vi "Update_Result_Table.vi"(7 "MCListbox Refnum":refnum<vi>, 9 "TempAnalysisResult":variant, 10 "ProjectName":string, 11 "Analysis Result":refnum<vi>) -> ()   [LabVIEW 2019]
uses:
  ROI/Controls/ROI_List_Action.ctl
  Analysis/Controls/Parttern Match/Analysis_PatternMatch_Parameter.ctl
  Analysis/Controls/Barcode 1D/Analysis_Barcode 1D_Parameter.ctl
  <vilib>/vision/Instrument.llb/Demodulation Mode.ctl
  <vilib>/vision/Instrument.llb/Cell Sample Size.ctl
  <vilib>/vision/Instrument.llb/Cell Filter Mode.ctl
  <vilib>/vision/Instrument.llb/QR Code Search Options.ctl
  <vilib>/vision/Instrument.llb/Data Matrix Polarity.ctl
  <vilib>/vision/Instrument.llb/QR Code Model Type.ctl
  <vilib>/vision/Instrument.llb/QR Code Description Options.ctl
  Analysis/Controls/Barcode 2D/Analysis_Barcode 2D_Parameter.ctl
  Analysis/Controls/Clamp MAX/Analysis_Clamp MAX_Parameter.ctl
  Analysis/Controls/Clamp/Analysis_Clamp_Parameter.ctl
  Analysis/Controls/Edge Detection/Analysis_Edge Detection_Parameter.ctl
  Analysis/Controls/Find Straight Edge/Analysis_Find Straight Edge_Parameter.ctl
  <vilib>/vision/Measure.llb/Straight Edge Process.ctl
  <vilib>/vision/Measure.llb/Straight Edge Options.ctl
  <vilib>/vision/Measure.llb/Edge Polarity.ctl
  <vilib>/vision/Measure.llb/Edge Options.ctl
  <vilib>/vision/Instrument.llb/Data Matrix Search Options.ctl
  <vilib>/vision/Instrument.llb/Data Matrix Mirror.ctl
  <vilib>/vision/Instrument.llb/Cell Fill Percentage.ctl
  <vilib>/vision/Instrument.llb/ECC Type.ctl
  <vilib>/vision/Instrument.llb/Data Matrix Description Options.ctl
  Analysis/Controls/Particle/Analysis_Particle_Parameter.ctl
  Analysis/Controls/Histogram/Analysis_Histogram_Parameter.ctl
  Analysis/Controls/Circle/Analysis_Circle_Parameter.ctl
  Analysis/Controls/ShapeDectect/Analysis_ShapeDectect_Parameter.ctl
  Analysis/Controls/OCR/Analysis_OCR_Setting Parameter.ctl
  Analysis/Controls/ColorMatch/Analysis_ColorMatch_Parameter.ctl
  <vilib>/vision/Instrument.llb/Data Matrix Advanced Options.ctl
  <vilib>/vision/Instrument.llb/Data Matrix Size Options.ctl
panel:
  in  "Selected Particle Report":T1(array[cluster])=[{"Area"=25.0, "Number of Holes"=0.0, "Bounding Rect"={"Left"=86.0, "Top"=0.0, "Right"=95.0, "Bottom"=7.0}, "Center of Mass"={"X"=89.88, "Y"=2.56}, "Orientation"=35.64802944169076, "Dimensions"={"Width"=9.0, "Height"=7.0}}, {"Area"=86262.0, "Number of Holes"=23.0, "Bounding Rect"={"Left"=0.0, "Top"=0.0, "Right"=463.0, "Bottom"=400.0}, "Center of Mass"={"X"=231.6348565996615, "Y"=215.4975423709165}, "Orientation"=163.33264135410136, "Dimensions"={"Width"=463.0, "Height"=400.0}}, {"Area"=1.0, "Number of Holes"=0.0, "Bounding Rect"={"Left"=412.0, "Top"=1.0, "Right"=413.0, "Bottom"=2.0}, "Center of Mass"={"X"=412.0, "Y"=1.0}, "Orientation"=-0.0, "Dimensions"={"Width"=1.0, "Height"=1.0}}, {"Area"=764.0, "Number of Holes"=1.0, "Bounding Rect"={"Left"=400.0, "Top"=1.0, "Right"=429.0, "Bottom"=38.0}, "Center of Mass"={"X"=414.1609947643979, "Y"=19.994764397905758}, "Orientation"=91.15464026101695, "Dimensions"={"Width"=29.0, "Height"=37.0}}, {"Area"=59.0, "Number of Holes"=0.0, "Bounding Rect"={"Left"=310.0, "Top"=6.0, "Right"=340.0, "Bottom"=29.0}, "Center of Mass"={"X"=326.50847457627117, "Y"=15.610169491525424}, "Orientation"=141.9692279302436, "Dimensions"={"Width"=30.0, "Height"=23.0}}, {"Area"=11.0, "Number of Holes"=0.0, "Bounding Rect"={"Left"=0.0, "Top"=7.0, "Right"=8.0, "Bottom"=12.0}, "Center of Mass"={"X"=3.090909090909091, "Y"=9.0}, "Orientation"=154.0962999034186, "Dimensions"={"Width"=8.0, "Height"=5.0}}, {"Area"=8.0, "Number of Holes"=0.0, "Bounding Rect"={"Left"=10.0, "Top"=12.0, "Right"=18.0, "Bottom"=15.0}, "Center of Mass"={"X"=13.5, "Y"=13.125}, "Orientation"=161.9863133074482, "Dimensions"={"Width"=8.0, "Height"=3.0}}, {"Area"=2191.0, "Number of Holes"=0.0, "Bounding Rect"={"Left"=108.0, "Top"=12.0, "Right"=160.0, "Bottom"=73.0}, "Center of Mass"={"X"=132.4596074851666, "Y"=44.30716567777271}, "Orientation"=94.97370367521454, "Dimensions"={"Width"=52.0, "Height"=61.0}}, {"Area"=18.0, "Number of Holes"=0.0, "Bounding Rect"={"Left"=136.0, "Top"=12.0, "Right"=150.0, "Bottom"=18.0}, "Center of Mass"={"X"=142.94444444444446, "Y"=13.833333333333334}, "Orientation"=159.1562056734768, "Dimensions"={"Width"=14.0, "Height"=6.0}}, {"Area"=4659.0, "Number of Holes"=2.0, "Bounding Rect"={"Left"=266.0, "Top"=12.0, "Right"=345.0, "Bottom"=101.0}, "Center of Mass"={"X"=303.5157759175789, "Y"=58.89869070616012}, "Orientation"=93.68626534635163, "Dimensions"={"Width"=79.0, "Height"=89.0}}, {"Area"=12.0, "Number of Holes"=0.0, "Bounding Rect"={"Left"=19.0, "Top"=14.0, "Right"=29.0, "Bottom"=17.0}, "Center of Mass"={"X"=23.083333333333332, "Y"=15.416666666666666}, "Orientation"=169.41797481154816, "Dimensions"={"Width"=10.0, "Height"=3.0}}, {"Area"=6.0, "Number of Holes"=0.0, "Bounding Rect"={"Left"=32.0, "Top"=17.0, "Right"=38.0, "Bottom"=18.0}, "Center of Mass"={"X"=34.5, "Y"=17.0}, "Orientation"=-0.0, "Dimensions"={"Width"=6.0, "Height"=1.0}}, {"Area"=1.0, "Number of Holes"=0.0, "Bounding Rect"={"Left"=40.0, "Top"=17.0, "Right"=41.0, "Bottom"=18.0}, "Center of Mass"={"X"=40.0, "Y"=17.0}, "Orientation"=-0.0, "Dimensions"={"Width"=1.0, "Height"=1.0}}, {"Area"=1.0, "Number of Holes"=0.0, "Bounding Rect"={"Left"=326.0, "Top"=23.0, "Right"=327.0, "Bottom"=24.0}, "Center of Mass"={"X"=326.0, "Y"=23.0}, "Orientation"=-0.0, "Dimensions"={"Width"=1.0, "Height"=1.0}}, {"Area"=72.0, "Number of Holes"=2.0, "Bounding Rect"={"Left"=388.0, "Top"=35.0, "Right"=410.0, "Bottom"=55.0}, "Center of Mass"={"X"=397.8888888888889, "Y"=46.52777777777778}, "Orientation"=136.8853757704328, "Dimensions"={"Width"=22.0, "Height"=20.0}}, {"Area"=2.0, "Number of Holes"=0.0, "Bounding Rect"={"Left"=342.0, "Top"=36.0, "Right"=343.0, "Bottom"=38.0}, "Center of Mass"={"X"=342.0, "Y"=36.5}, "Orientation"=90.0, "Dimensions"={"Width"=1.0, "Height"=2.0}}, {"Area"=1.0, "Number of Holes"=0.0, "Bounding Rect"={"Left"=396.0, "Top"=49.0, "Right"=397.0, "Bottom"=50.0}, "Center of Mass"={"X"=396.0, "Y"=49.0}, "Orientation"=-0.0, "Dimensions"={"Width"=1.0, "Height"=1.0}}, {"Area"=2.0, "Number of Holes"=0.0, "Bounding Rect"={"Left"=411.0, "Top"=54.0, "Right"=413.0, "Bottom"=55.0}, "Center of Mass"={"X"=411.5, "Y"=54.0}, "Orientation"=-0.0, "Dimensions"={"Width"=2.0, "Height"=1.0}}, {"Area"=86.0, "Number of Holes"=0.0, "Bounding Rect"={"Left"=457.0, "Top"=74.0, "Right"=463.0, "Bottom"=96.0}, "Center of Mass"={"X"=460.2674418604651, "Y"=84.55813953488372}, "Orientation"=89.65892383367937, "Dimensions"={"Width"=6.0, "Height"=22.0}}, {"Area"=1300.0, "Number of Holes"=0.0, "Bounding Rect"={"Left"=30.0, "Top"=82.0, "Right"=67.0, "Bottom"=127.0}, "Center of Mass"={"X"=48.050769230769234, "Y"=104.12153846153846}, "Orientation"=84.17144755534598, "Dimensions"={"Width"=37.0, "Height"=45.0}}, {"Area"=1.0, "Number of Holes"=0.0, "Bounding Rect"={"Left"=450.0, "Top"=105.0, "Right"=451.0, "Bottom"=106.0}, "Center of Mass"={"X"=450.0, "Y"=105.0}, "Orientation"=-0.0, "Dimensions"={"Width"=1.0, "Height"=1.0}}, {"Area"=3.0, "Number of Holes"=0.0, "Bounding Rect"={"Left"=243.0, "Top"=124.0, "Right"=245.0, "Bottom"=126.0}, "Center of Mass"={"X"=243.66666666666666, "Y"=124.33333333333333}, "Orientation"=135.00000000000014, "Dimensions"={"Width"=2.0, "Height"=2.0}}, {"Area"=28.0, "Number of Holes"=0.0, "Bounding Rect"={"Left"=271.0, "Top"=127.0, "Right"=293.0, "Bottom"=136.0}, "Center of Mass"={"X"=281.39285714285717, "Y"=131.39285714285714}, "Orientation"=158.88118737593115, "Dimensions"={"Width"=22.0, "Height"=9.0}}, {"Area"=4.0, "Number of Holes"=0.0, "Bounding Rect"={"Left"=250.0, "Top"=128.0, "Right"=253.0, "Bottom"=130.0}, "Center of Mass"={"X"=251.0, "Y"=128.5}, "Orientation"=148.282525588539, "Dimensions"={"Width"=3.0, "Height"=2.0}}, {"Area"=4.0, "Number of Holes"=0.0, "Bounding Rect"={"Left"=255.0, "Top"=132.0, "Right"=258.0, "Bottom"=134.0}, "Center of Mass"={"X"=256.0, "Y"=132.5}, "Orientation"=148.282525588539, "Dimensions"={"Width"=3.0, "Height"=2.0}}, {"Area"=2.0, "Number of Holes"=0.0, "Bounding Rect"={"Left"=260.0, "Top"=136.0, "Right"=262.0, "Bottom"=138.0}, "Center of Mass"={"X"=260.5, "Y"=136.5}, "Orientation"=135.0, "Dimensions"={"Width"=2.0, "Height"=2.0}}, {"Area"=1.0, "Number of Holes"=0.0, "Bounding Rect"={"Left"=300.0, "Top"=136.0, "Right"=301.0, "Bottom"=137.0}, "Center of Mass"={"X"=300.0, "Y"=136.0}, "Orientation"=-0.0, "Dimensions"={"Width"=1.0, "Height"=1.0}}, {"Area"=6.0, "Number of Holes"=0.0, "Bounding Rect"={"Left"=263.0, "Top"=139.0, "Right"=269.0, "Bottom"=145.0}, "Center of Mass"={"X"=265.5, "Y"=141.5}, "Orientation"=135.0, "Dimensions"={"Width"=6.0, "Height"=6.0}}, {"Area"=4.0, "Number of Holes"=0.0, "Bounding Rect"={"Left"=296.0, "Top"=139.0, "Right"=299.0, "Bottom"=141.0}, "Center of Mass"={"X"=297.25, "Y"=139.25}, "Orientation"=161.56505117707798, "Dimensions"={"Width"=3.0, "Height"=2.0}}, {"Area"=1.0, "Number of Holes"=0.0, "Bounding Rect"={"Left"=269.0, "Top"=146.0, "Right"=270.0, "Bottom"=147.0}, "Center of Mass"={"X"=269.0, "Y"=146.0}, "Orientation"=-0.0, "Dimensions"={"Width"=1.0, "Height"=1.0}}, {"Area"=3.0, "Number of Holes"=0.0, "Bounding Rect"={"Left"=271.0, "Top"=148.0, "Right"=273.0, "Bottom"=151.0}, "Center of Mass"={"X"=271.3333333333333, "Y"=149.0}, "Orientation"=118.15496623701016, "Dimensions"={"Width"=2.0, "Height"=3.0}}, {"Area"=2795.0, "Number of Holes"=2.0, "Bounding Rect"={"Left"=375.0, "Top"=149.0, "Right"=427.0, "Bottom"=220.0}, "Center of Mass"={"X"=400.8608228980322, "Y"=184.37352415026834}, "Orientation"=84.46336335814708, "Dimensions"={"Width"=52.0, "Height"=71.0}}, {"Area"=6024.0, "Number of Holes"=9.0, "Bounding Rect"={"Left"=176.0, "Top"=152.0, "Right"=254.0, "Bottom"=252.0}, "Center of Mass"={"X"=211.63097609561754, "Y"=201.42861885790174}, "Orientation"=84.84991716022375, "Dimensions"={"Width"=78.0, "Height"=100.0}}, {"Area"=1.0, "Number of Holes"=0.0, "Bounding Rect"={"Left"=275.0, "Top"=154.0, "Right"=276.0, "Bottom"=155.0}, "Center of Mass"={"X"=275.0, "Y"=154.0}, "Orientation"=-0.0, "Dimensions"={"Width"=1.0, "Height"=1.0}}, {"Area"=2.0, "Number of Holes"=0.0, "Bounding Rect"={"Left"=462.0, "Top"=209.0, "Right"=463.0, "Bottom"=211.0}, "Center of Mass"={"X"=462.0, "Y"=209.5}, "Orientation"=90.0, "Dimensions"={"Width"=1.0, "Height"=2.0}}, {"Area"=1.0, "Number of Holes"=0.0, "Bounding Rect"={"Left"=460.0, "Top"=214.0, "Right"=461.0, "Bottom"=215.0}, "Center of Mass"={"X"=460.0, "Y"=214.0}, "Orientation"=-0.0, "Dimensions"={"Width"=1.0, "Height"=1.0}}, {"Area"=2.0, "Number of Holes"=0.0, "Bounding Rect"={"Left"=459.0, "Top"=216.0, "Right"=460.0, "Bottom"=218.0}, "Center of Mass"={"X"=459.0, "Y"=216.5}, "Orientation"=90.0, "Dimensions"={"Width"=1.0, "Height"=2.0}}, {"Area"=3.0, "Number of Holes"=0.0, "Bounding Rect"={"Left"=249.0, "Top"=220.0, "Right"=251.0, "Bottom"=223.0}, "Center of Mass"={"X"=249.66666666666666, "Y"=221.0}, "Orientation"=61.84503376298985, "Dimensions"={"Width"=2.0, "Height"=3.0}}, {"Area"=1243.0, "Number of Holes"=2.0, "Bounding Rect"={"Left"=26.0, "Top"=222.0, "Right"=62.0, "Bottom"=266.0}, "Center of Mass"={"X"=43.17940466613033, "Y"=243.51729686242962}, "Orientation"=85.94368880614128, "Dimensions"={"Width"=36.0, "Height"=44.0}}, {"Area"=3.0, "Number of Holes"=0.0, "Bounding Rect"={"Left"=248.0, "Top"=224.0, "Right"=250.0, "Bottom"=227.0}, "Center of Mass"={"X"=248.33333333333334, "Y"=225.0}, "Orientation"=61.84503376298985, "Dimensions"={"Width"=2.0, "Height"=3.0}}, {"Area"=1.0, "Number of Holes"=0.0, "Bounding Rect"={"Left"=62.0, "Top"=237.0, "Right"=63.0, "Bottom"=238.0}, "Center of Mass"={"X"=62.0, "Y"=237.0}, "Orientation"=-0.0, "Dimensions"={"Width"=1.0, "Height"=1.0}}, {"Area"=1.0, "Number of Holes"=0.0, "Bounding Rect"={"Left"=63.0, "Top"=241.0, "Right"=64.0, "Bottom"=242.0}, "Center of Mass"={"X"=63.0, "Y"=241.0}, "Orientation"=-0.0, "Dimensions"={"Width"=1.0, "Height"=1.0}}, {"Area"=25.0, "Number of Holes"=0.0, "Bounding Rect"={"Left"=60.0, "Top"=277.0, "Right"=78.0, "Bottom"=285.0}, "Center of Mass"={"X"=68.52, "Y"=279.96}, "Orientation"=21.66201240397291, "Dimensions"={"Width"=18.0, "Height"=8.0}}, {"Area"=2.0, "Number of Holes"=0.0, "Bounding Rect"={"Left"=57.0, "Top"=285.0, "Right"=59.0, "Bottom"=287.0}, "Center of Mass"={"X"=57.5, "Y"=285.5}, "Orientation"=45.0, "Dimensions"={"Width"=2.0, "Height"=2.0}}, {"Area"=1575.0, "Number of Holes"=0.0, "Bounding Rect"={"Left"=302.0, "Top"=285.0, "Right"=345.0, "Bottom"=337.0}, "Center of Mass"={"X"=321.4095238095238, "Y"=308.74603174603175}, "Orientation"=73.7943685874199, "Dimensions"={"Width"=43.0, "Height"=52.0}}, {"Area"=4853.0, "Number of Holes"=6.0, "Bounding Rect"={"Left"=54.0, "Top"=304.0, "Right"=130.0, "Bottom"=388.0}, "Center of Mass"={"X"=91.93962497424273, "Y"=344.35854110859265}, "Orientation"=86.14198788768665, "Dimensions"={"Width"=76.0, "Height"=84.0}}, {"Area"=28.0, "Number of Holes"=0.0, "Bounding Rect"={"Left"=323.0, "Top"=332.0, "Right"=338.0, "Bottom"=341.0}, "Center of Mass"={"X"=330.57142857142856, "Y"=336.64285714285717}, "Orientation"=29.47782205630064, "Dimensions"={"Width"=15.0, "Height"=9.0}}, {"Area"=3.0, "Number of Holes"=0.0, "Bounding Rect"={"Left"=312.0, "Top"=366.0, "Right"=315.0, "Bottom"=367.0}, "Center of Mass"={"X"=313.0, "Y"=366.0}, "Orientation"=-0.0, "Dimensions"={"Width"=3.0, "Height"=1.0}}, {"Area"=1.0, "Number of Holes"=0.0, "Bounding Rect"={"Left"=436.0, "Top"=396.0, "Right"=437.0, "Bottom"=397.0}, "Center of Mass"={"X"=436.0, "Y"=396.0}, "Orientation"=-0.0, "Dimensions"={"Width"=1.0, "Height"=1.0}}, {"Area"=1.0, "Number of Holes"=0.0, "Bounding Rect"={"Left"=434.0, "Top"=397.0, "Right"=435.0, "Bottom"=398.0}, "Center of Mass"={"X"=434.0, "Y"=397.0}, "Orientation"=-0.0, "Dimensions"={"Width"=1.0, "Height"=1.0}}, {"Area"=36.0, "Number of Holes"=0.0, "Bounding Rect"={"Left"=318.0, "Top"=398.0, "Right"=340.0, "Bottom"=400.0}, "Center of Mass"={"X"=328.5, "Y"=398.6111111111111}, "Orientation"=-0.0, "Dimensions"={"Width"=22.0, "Height"=2.0}}, {"Area"=8.0, "Number of Holes"=0.0, "Bounding Rect"={"Left"=427.0, "Top"=398.0, "Right"=433.0, "Bottom"=400.0}, "Center of Mass"={"X"=429.75, "Y"=398.625}, "Orientation"=11.525650458236512, "Dimensions"={"Width"=6.0, "Height"=2.0}}]
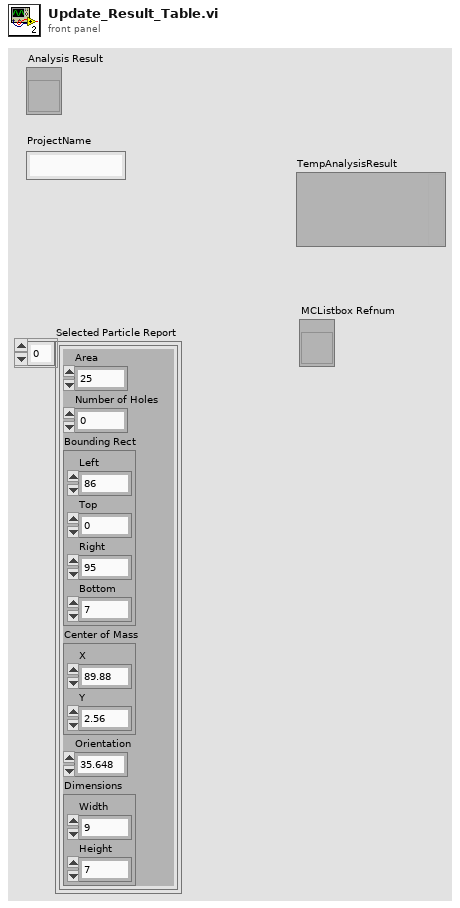
[diagram p1: front panel]
types:
  T1 = cluster{"Area":dbl, "Number of Holes":dbl, "Bounding Rect":cluster{"Left":dbl, "Top":dbl, "Right":dbl, "Bottom":dbl}, "Center of Mass":cluster{"X":dbl, "Y":dbl}, "Orientation":dbl, "Dimensions":cluster{"Width":dbl, "Height":dbl}}[]
  T2 = typedef "ROI_List_Action.ctl" = enum16{"Init", "Add ROI", "Delete ROI", "Get All ROI", "Get Specific ROI", "Set Analysis Setting", "Set Process Setting", "Replace All Entries", "ROIEntryBackup", "ROIEntryBackupClear", "ROIEntryReturn"}
  T3 = typedef "Vision_DataEntry.ctl" = cluster{"vROIName":string, "vROIContour":cluster{"Contour Type":u32, "ROI Type":u32, "Points":i32[]}, "ProcessSetting":T4[], "Analysis_Setting":T6}
  T4 = typedef "Process_Setting.ctl" = cluster{"Enum_PreProcess":T5, "Parameter":string}
  T5 = typedef "VisionProcessName.ctl" = enum16{"*CamParameter*", "CamAttributes", "*Preprocess*", "CG_Brightness", "C_Plane Extraction", "C_Threshold", "G_Lookup Table", "G_Threshold"}
  T6 = typedef "Analysis_Setting.ctl" = cluster{"PreProcess":T7, "Parameter":string}
  T7 = typedef "V_Analysis_Type.ctl" = enum16{"None", "C_Color Pattern Matching", "G_PatternMatching", "G_ShapeDectect", "G_GeometricMatch", "B_Area Check"}
  T8 = typedef "ROI Descriptor" = cluster{"Global Rectangle":i32[], "Contours":cluster{"ID":enum32{"External", "Internal"}, "Type":u32, "Coordinates":i32[]}[]}
  T9 = cluster{"Algorithm":i32, "Match Parameters":cluster{"Number of Matches Requested":i32, "Minimum Match Score":sgl, "Angle Ranges":cluster{"Start Angle":sgl, "End Angle":sgl}[]}, "ROI Descriptor":T8, "Advanced Options":cluster{"Item":u16, "Value":dbl}[], "Template path":string}
  T10 = typedef "Analysis_Circle_Parameter.ctl" = cluster{"ROI Descriptor":cluster{"Global Rectangle":i32[], "Contours":cluster{"Contour Type":u32, "ROI Type":u32, "Points":i32[]}[]}, "Options":cluster{"Search  Direction":u32, "Edge Options":T11, "Show Search Area":bool, "Show Search Lines":bool, "Show Edges Found":bool, "Show Result":bool, "Search Area Color":u32, "Search Lines Color":u32, "Edge Locations Color":u32, "Result Color":u32, "Overlay Group Name":string}, "Circle Fit Options":cluster{"Process":enum16{"Get First Edge", "Get First + Last Edge", "Get All Edges", "Get Best Edge"}, "Step Size":dbl, "Max Pixel Radius":i32}}
  T11 = typedef "Edge Options.ctl" = cluster{"Edge Polarity":T12, "Kernel Size":u32, "Width":u32, "Minimum Edge Strength":sgl, "Interpolation Type":enum32{"Zero Order", "Bilinear", "Quadratic", "Cubic", "Bilinear Fixed"}, "Data Processing Method":enum32{"Average", "Median"}}
  T12 = typedef "Edge Polarity.ctl" = u32
  T13 = typedef "Analysis_ShapeDectect_Parameter.ctl" = cluster{"Enum_ShapeType":enum16{"Circles", "Ellipses", "Lines", "Rectangles"}, "MaxParticle":i32, "Descriptor":cluster{"Set 1":dbl, "Set 2":dbl, "Set 3":dbl, "Set 4":dbl}, "Match Options":cluster{"Rotation":bool, "Scale":bool, "Occlusion":bool, "Range Settings":cluster{"Match Constraints":u32, "Min":dbl, "Max":dbl}[]}, "Curve Parameters":cluster{"Extraction Mode":u32, "Edge Threshold":i32, "Edge Filter Size":u32, "Min Length":i32, "Row Search Step Size":i32, "Col Search Step Size":i32, "Max Endpoint Gap":i32, "Closed":bool, "Subpixel":bool}, " score":dbl}
  T14 = typedef "Analysis_OCR_Setting Parameter.ctl" = cluster{"OCRSelectedLanaguage":string[]}
  T15 = typedef "Analysis_ColorMatch_Parameter.ctl" = cluster{"Color Sensitivity":u32, "Learn Saturation Threshold":i32, "Minimum Match Score":dbl, "Match Saturation Threshold":i32, "ROI Descriptor":T8, "TemplatePath":string, "ColorSpectrum":dbl[]}
  T16 = typedef "Analysis_Type.ctl" = u16
  T17 = typedef "Analysis_PatternMatch_Parameter.ctl" = cluster{"Algorithm":i32, "Match Parameters":cluster{"Number of Matches Requested":i32, "Minimum Match Score":sgl, "Angle Ranges":cluster{"Start Angle":sgl, "End Angle":sgl}[]}, "ROI Descriptor":T8, "Advanced Options":cluster{"Item":u16, "Value":dbl}[], "Template path":string, "XOffset":i32, "YOffset":i32}
  T18 = cluster{"Number of Matches Requested":i32, "Minimum Match Score":sgl, "Angle Ranges":cluster{"Start Angle":sgl, "End Angle":sgl}[]}
  T19 = typedef "Analysis_Edge Detection_Parameter.ctl" = cluster{"Edge Options":cluster{"Edge Polarity":u16, "Kernel Size":u32, "Width":u32, "Minimum Edge Strength":dbl, "Interpolation Type":u16, "Data Processing Method":u16}, "Process":u16, "Number of Matches Requested":i32, "ROI Descriptor":cluster{"Global Rectangle":i32[], "Contours":cluster{"Contour Type":u32, "ROI Type":u32, "Points":i32[]}[]}}
  T20 = typedef "Analysis_Barcode 1D_Parameter.ctl" = cluster{"Barcode Search Options":cluster{"Min Bar Width":dbl, "Min Edge Strength":dbl, "Min Bars":dbl, "Skip Location Search?":bool}, "Barcode Types To Search":enum16{"Reserved", "Codabar", "Code 39", "Code 93", "Code 128", "EAN 8", "EAN 13", "Interleaved 2 of 5", "MSI", "UPCA", "Pharmacode", "RSS Limited"}[], "Barcode Grading Options":cluster{"Calculate Grading Report":bool, "Scan Width ":dbl}, "Number of Matches Requested":i32, "ROI":cluster{"Global Rectangle":i32[], "Contours":cluster{"Contour Type":u32, "ROI Type":u32, "Points":i32[]}[]}}
  T21 = typedef "Analysis_Barcode 2D_Parameter.ctl" = cluster{"ROI":cluster{"Global Rectangle":i32[], "Contours":cluster{"Contour Type":u32, "ROI Type":u32, "Points":i32[]}[]}, "Barcode Type":enum16{"Data Matrix", "PDF417", "QR Code"}, "Data Matrix Parameter":cluster{"Data Matrix Description Options":T22, "Data Matrix Search Options":T27, "Data Matrix Size Options":T31, "Advanced Options":T32[]}, "PDF147 Search Mode":T33, "QR Code Parameter":cluster{"QR Search Options":T34, "QR Description Options":T35, "QR Code Cell Size (pixels)":cluster{"Minimum Size":u32, "Maximum Size":u32}}}
  T22 = typedef "Data Matrix Description Options.ctl" = cluster{"Aspect Ratio":sgl, "Rows":u32, "Columns":u32, "Rectangle":bool, "ECC":T23, "Barcode Polarity":T24, "Cell Fill Percentage":T25, "Minimum Border Integrity %":sgl, "Mirror Mode":T26}
  T23 = typedef "ECC Type.ctl" = i32
  T24 = typedef "Data Matrix Polarity.ctl" = i32
  T25 = typedef "Cell Fill Percentage.ctl" = i32
  T26 = typedef "Data Matrix Mirror.ctl" = i32
  T27 = typedef "Data Matrix Search Options.ctl" = cluster{"Rotation Mode":enum32{"Unlimited", "0 Degrees", "90 Degrees", "180 Degrees", "270 Degrees"}, "Skip Location?":bool, "Edge Threshold":u32, "Demodulation Mode":T28, "Cell Sample Size":T29, "Cell Filter Mode":T30, "Skew Degrees Allowed":u32, "Maximum Iterations":u32, "Initial Search Vector Width":u32}
  T28 = typedef "Demodulation Mode.ctl" = i32
  T29 = typedef "Cell Sample Size.ctl" = i32
  T30 = typedef "Cell Filter Mode.ctl" = i32
  T31 = typedef "Data Matrix Size Options.ctl" = cluster{"Data Matrix Size":cluster{"Minimum Size":u32, "Maximum Size":u32}, "Quiet Zone Width":u32}
  T32 = typedef "Data Matrix Advanced Options.ctl" = cluster{"Option":enum32{"Line Detection", "HighLight Filter", "Aggressive", "FNC1", "Refine Bounding Box"}, " Value":dbl}
  T33 = typedef "PDF417 Search Mode" = enum32{"Multiple Barcodes", "Single Barcode, Conservative"}
  T34 = typedef "QR Code Search Options.ctl" = cluster{"Rotation Mode":enum32{"Unlimited", "0 Degrees", "90 Degrees", "180 Degrees", "270 Degrees"}, "Skip Location?":bool, "Edge Threshold":u32, "Demodulation Mode":T28, "Cell Sample Size":T29, "Cell Filter Mode":T30, "Skew Degrees Allowed":u32}
  T35 = typedef "QR Code Description Options.ctl" = cluster{"Matrix Size (cells)":i32, "Barcode Polarity":T24, "Mirror Mode":i32, "QR Model":T36}
  T36 = typedef "QR Code Model Type.ctl" = i32
  T37 = typedef "Analysis_Clamp_Parameter.ctl" = cluster{"Clamp Settings":cluster{"Contrast":i32, "Filter width":i32, "Steepness":i32, "Subsampling Ratio":u32, "Show Search Area":bool, "Show Search Lines":bool, "Show Edges Found":bool, "Show Result":bool}, "ROI Descriptor":cluster{"Global Rectangle":i32[], "Contours":cluster{"Contour Type":u32, "ROI Type":u32, "Points":i32[]}[]}, "Process":u16}
  T38 = typedef "Analysis_Clamp MAX_Parameter.ctl" = cluster{"Overlay Settings":cluster{"Show Search Area":bool, "Show Curves":bool, "Show Clamp Locations":bool, "Show Result":bool, "Search Area Color":u32, "Curves Color":u32, "Clamp Locations Color":u32, "Result Color":u32, "Overlay Group Name":string}, "Curve Extraction Settings":cluster{"Extraction Mode":u32, "Edge Threshold":i32, "Edge Filter Size":u32, "Min Length":i32, "Row Search Step Size":i32, "Col Search Step Size":i32, "Max Endpoint Gap":i32, "Closed":bool, "Subpixel":bool}, "Clamp Settings":cluster{"Angle Range (+/-)":dbl, "Edge Polarity":cluster{"Start":u32, "End":u32}}, "ROI":cluster{"Global Rectangle":i32[], "Contours":cluster{"Contour Type":u32, "ROI Type":u32, "Points":i32[]}[]}}
  T39 = typedef "Analysis_Particle_Parameter.ctl" = cluster{"Selected Particle":i32, "Connectivity 4/8 (8)":bool, "MaxParticle":i32}
  T40 = typedef "Analysis_Histogram_Parameter.ctl" = cluster{"Interval Range":cluster{"Minimum":sgl, "Maximum":sgl}, "ROI Out":cluster{"Global Rectangle":i32[], "Contours":cluster{"Contour Type":u32, "ROI Type":u32, "Points":i32[]}[]}, "Number of Classes":i32}
  T41 = typedef "Analysis_Find Straight Edge_Parameter.ctl" = cluster{"ROI Descriptor":cluster{"Global Rectangle":i32[], "Contours":cluster{"Contour Type":u32, "ROI Type":u32, "Points":i32[]}[]}, "Number of Matches Requested":i32, "Edge Info Size":i32, "Options":cluster{"Search Direction":u32, "Edge Options":T11, "Show Search Area":bool, "Show Search Lines":bool, "Show Edges Found":bool, "Show Result":bool, "Search Area Color":u32, "Search Lines Color":u32, "Edge Locations Color":u32, "Result Color":u32, "Overlay Group Name":string}, "Line Fit Options":T42}
  T42 = typedef "Straight Edge Options.ctl" = cluster{"Number of Lines":i32, "Type":T43, "Min. Score":dbl, "Max. Score":dbl, "Orientation":dbl, "Angle Range":dbl, "Angle Tolerance":dbl, "Step Size":u32, "Min. SNR (db)":dbl, "Min. Points (%)":dbl, "Hough Iterations":i32}
  T43 = typedef "Straight Edge Process.ctl" = enum32{"First Edge Rake", "Best Edge Rake", "Hough Edge Rake", "First Edge Projection", "Best Edge Projection"}
  T44 = cluster{"ID":enum32{"External", "Internal"}, "Type":u32, "Coordinates":i32[]}[]
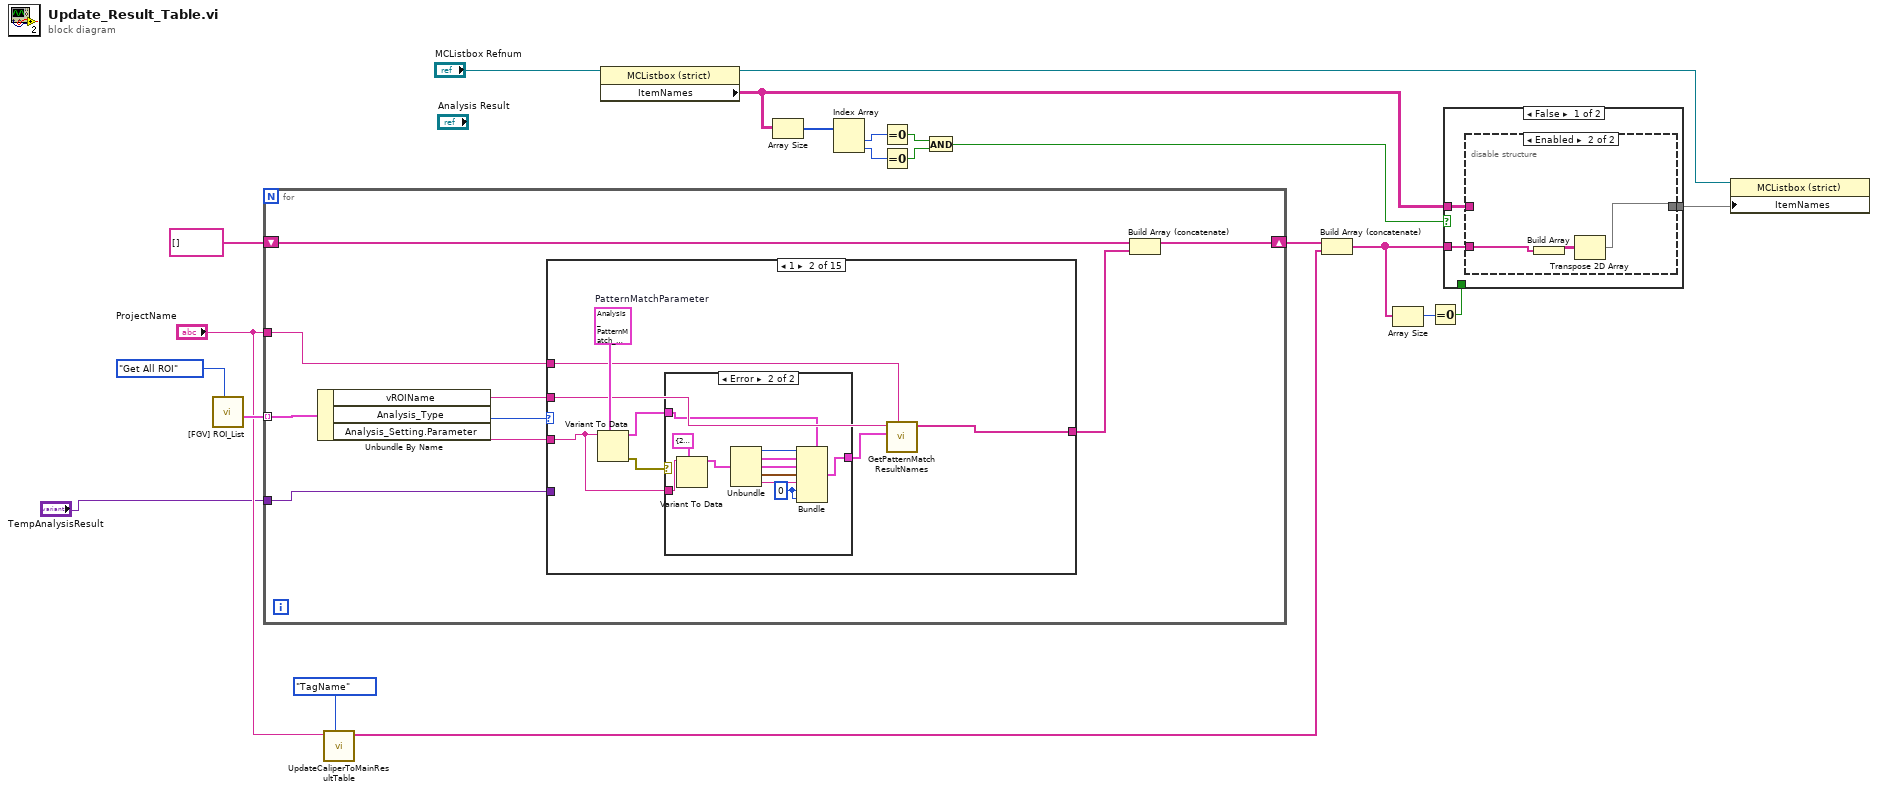
[diagram p0: block diagram]
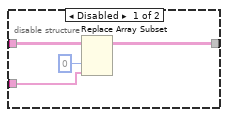
[diagram p2: hidden frame]
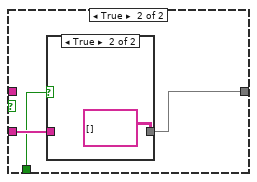
[diagram p3: hidden frame]
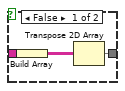
[diagram p4: hidden frame]
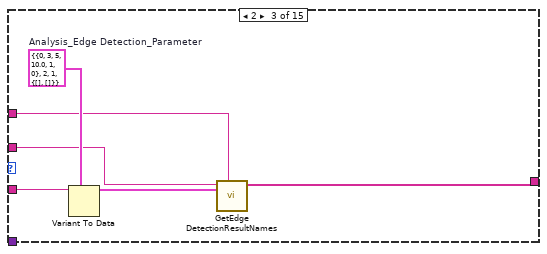
[diagram p7: hidden frame]
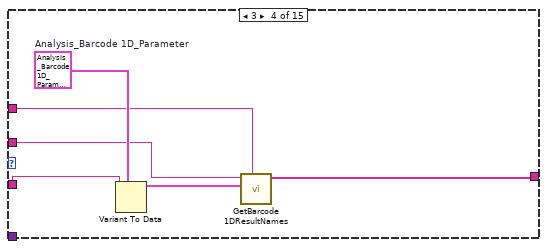
[diagram p8: hidden frame]
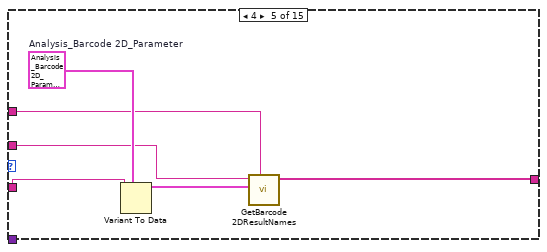
[diagram p9: hidden frame]
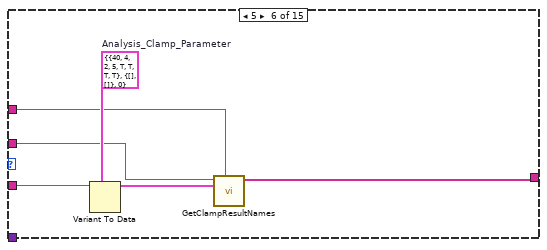
[diagram p10: hidden frame]
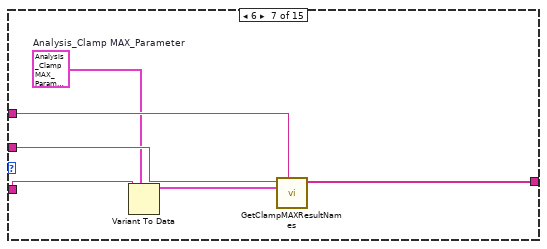
[diagram p11: hidden frame]
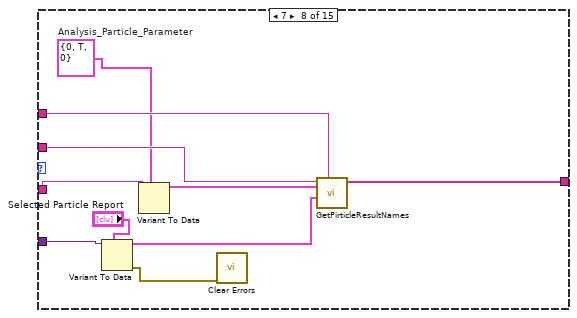
[diagram p12: hidden frame]
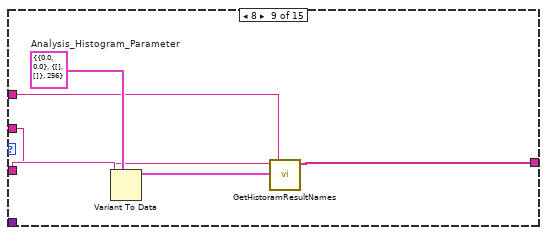
[diagram p13: hidden frame]
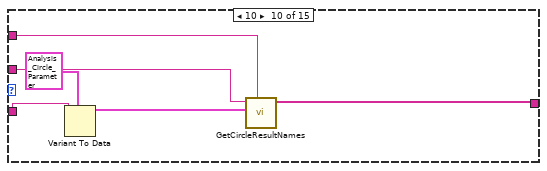
[diagram p14: hidden frame]
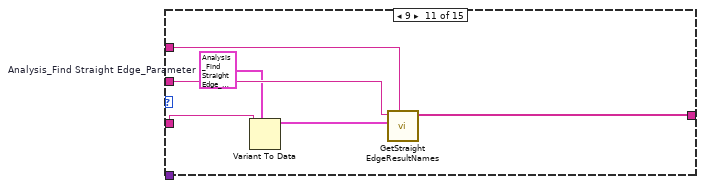
[diagram p15: hidden frame]
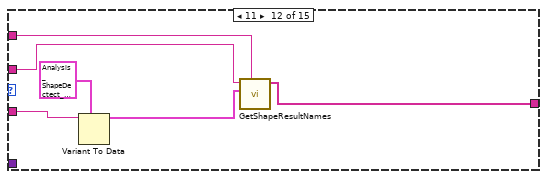
[diagram p16: hidden frame]
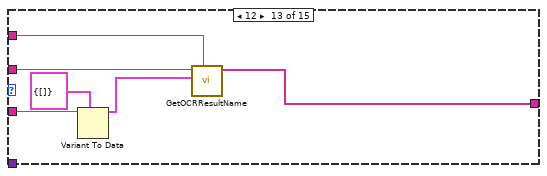
[diagram p17: hidden frame]
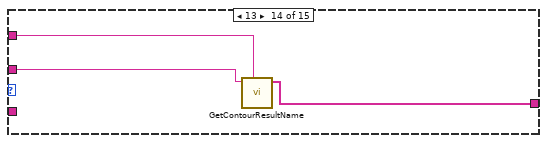
[diagram p18: hidden frame]
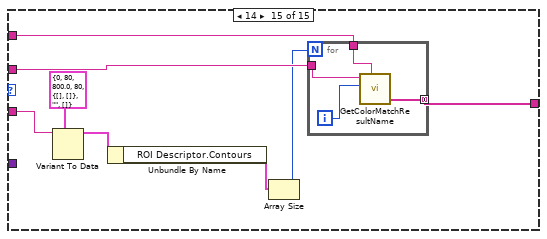
[diagram p19: hidden frame]
diagram:
  n1 = call "[FGV] ROI_List.vi"("Action"=ROI_List_Action."Get All ROI") -> ("All ROI"=w20:T3[])  [unwired: 8 in, 2 out]
  n2 = for {
    tunnel: w20 -> [w30] mode=indexing
    shift-right: [w25] -> w5
    shift-left: string[] [] -> [w26]
    tunnel: "ProjectName" -> [w23]
    tunnel: "TempAnalysisResult" -> [w22]
    n3 = Unbundle By Name(w30) -> ("vROIName"=w27:string, "Analysis_Type"=w29:T16, "Analysis_Setting.Parameter"=w28:string)
    n4 = case shown="1" w29 {
      tunnel: w28 -> [_ w34 w56 w62 w68 w74 w80 w90 w96 w102 w108 w114 w118 _ w127]
      tunnel: w27 -> [_ w37 w53 w58 w65 w71 w78 w88 w92 w99 w107 w112 w119 w123 w131]
      tunnel: w23 -> [_ w36 w54 w59 w66 w72 w79 w89 w94 w100 w105 w113 w120 w122 w130]
      tunnel: [_ w35 w51 w57 w63 w69 w77 w87 w93 w97 w106 w109 w115 w121 w129] -> w24
      tunnel: w22 -> [_ _ _ _ _ _ _ w84 _ _ _ _ _ _ _]
      frame 0, Default {
      }
      frame 1 {
        w38 = T17 {"Algorithm"=2, "Match Parameters"={"Number of Matches Requested"=1, "Minimum Match Score"=750.0, "Angle Ranges"=[]}, "ROI Descriptor"={"Global Rectangle"=[], "Contours"=[]}, "Advanced Options"=[{"Item"=1, "Value"=1.0}, {"Item"=103, "Value"=1.0}], "Template path"="", "XOffset"=0, "YOffset"=0}  # PatternMatchParameter
        n5 = Variant To Data(type=w38, Variant=w34) -> (data=w32:T17, error out=w33:errorcluster)  [unwired: 1 in]
        n6 = case shown="Error" w33 {
          tunnel: w34 -> [_ w49]
          tunnel: [w39 w47] -> w31
          tunnel: w32 -> [w39 w48]
          frame No Error {
          }
          frame Error {
            w40 = 0 ("XOffset")
            n7 = Variant To Data(type=T9 {"Algorithm"=2, "Match Parameters"={"Number of Matches Requested"=1, "Minimum Match Score"=750.0, "Angle Ranges"=[]}, "ROI Descriptor"={"Global Rectangle"=[], "Contours"=[]}, "Advanced Options"=[{"Item"=1, "Value"=1.0}, {"Item"=103, "Value"=1.0}], "Template path"=""} ("PatternMatchParameter"), Variant=w49) -> (data=w46:T9)  [unwired: 1 in, 1 out]
            n8 = Unbundle(w46) -> ("Algorithm"=w45:i32, "Match Parameters"=w44:T18, "ROI Descriptor"=w43:T8, "Advanced Options"=w42:cluster{"Item":u16, "Value":dbl}[], "Template path"=w41:string)
            n9 = Bundle(cluster=w48, "Algorithm"=w45, "Match Parameters"=w44, "ROI Descriptor"=w43, "Advanced Options"=w42, "Template path"=w41, "XOffset"=w40, "YOffset"=w40) -> (w47:T17)
          }
        }
        n10 = call "GetPatternMatchResultNames.vi"("ProjectName"=w36, "PatternMatchParameter"=w31, "ROI_Name"=w37) -> ("ResultNames"=w35:string[])  [unwired: 7 in, 1 out]
      }
      frame 2 {
        w55 = T19 {"Edge Options"={"Edge Polarity"=0, "Kernel Size"=3, "Width"=5, "Minimum Edge Strength"=10.0, "Interpolation Type"=1, "Data Processing Method"=0}, "Process"=2, "Number of Matches Requested"=1, "ROI Descriptor"={"Global Rectangle"=[], "Contours"=[]}}  # Analysis_Edge Detection_Parameter
        n11 = Variant To Data(type=w55, Variant=w56) -> (data=w52:T19)  [unwired: 1 in, 1 out]
        n12 = call "GetEdge DetectionResultNames.vi"("ProjectName"=w54, "Analysis_Edge Detection_Parameter"=w52, "ROI_Name"=w53) -> ("ResultNames"=w51:string[])  [unwired: 8 in]
      }
      frame 3 {
        w61 = T20 {"Barcode Search Options"={"Min Bar Width"=0.0, "Min Edge Strength"=0.0, "Min Bars"=0.0, "Skip Location Search?"=FALSE}, "Barcode Types To Search"=[enum."EAN 13", enum."Code 128", enum."Code 39"], "Barcode Grading Options"={"Calculate Grading Report"=FALSE, "Scan Width "=0.0}, "Number of Matches Requested"=1, "ROI"={"Global Rectangle"=[], "Contours"=[]}}  # Analysis_Barcode 1D_Parameter
        n13 = Variant To Data(type=w61, Variant=w62) -> (data=w60:T20)  [unwired: 1 in, 1 out]
        n14 = call "GetBarcode 1DResultNames.vi"("ProjectName"=w59, "Analysis_Barcode 1D_Parameter"=w60, "ROI_Name"=w58) -> ("ResultNames"=w57:string[])  [unwired: 7 in, 1 out]
      }
      frame 4 {
        w67 = T21 {"ROI"={"Global Rectangle"=[], "Contours"=[]}, "Barcode Type"=enum."PDF417", "Data Matrix Parameter"={"Data Matrix Description Options"={"Aspect Ratio"=0.0, "Rows"=0, "Columns"=0, "Rectangle"=FALSE, "ECC"=-2, "Barcode Polarity"=0, "Cell Fill Percentage"=-2, "Minimum Border Integrity %"=80.0, "Mirror Mode"=-2}, "Data Matrix Search Options"={"Rotation Mode"=enum."Unlimited", "Skip Location?"=FALSE, "Edge Threshold"=30, "Demodulation Mode"=-2, "Cell Sample Size"=-2, "Cell Filter Mode"=-2, "Skew Degrees Allowed"=5, "Maximum Iterations"=500, "Initial Search Vector Width"=5}, "Data Matrix Size Options"={"Data Matrix Size"={"Minimum Size"=0, "Maximum Size"=0}, "Quiet Zone Width"=10}, "Advanced Options"=[]}, "PDF147 Search Mode"=enum."Multiple Barcodes", "QR Code Parameter"={"QR Search Options"={"Rotation Mode"=enum."Unlimited", "Skip Location?"=FALSE, "Edge Threshold"=30, "Demodulation Mode"=-2, "Cell Sample Size"=-2, "Cell Filter Mode"=-2, "Skew Degrees Allowed"=5}, "QR Description Options"={"Matrix Size (cells)"=0, "Barcode Polarity"=-2, "Mirror Mode"=-2, "QR Model"=0}, "QR Code Cell Size (pixels)"={"Minimum Size"=3, "Maximum Size"=7}}}  # Analysis_Barcode 2D_Parameter
        n15 = Variant To Data(type=w67, Variant=w68) -> (data=w64:T21)  [unwired: 1 in, 1 out]
        n16 = call "GetBarcode 2DResultNames.vi"("ProjectName"=w66, "data IN"=w64, "ROI_Name"=w65) -> ("ResultNames"=w63:string[])  [unwired: 8 in]
      }
      frame 5 {
        w73 = T37 {"Clamp Settings"={"Contrast"=40, "Filter width"=4, "Steepness"=2, "Subsampling Ratio"=5, "Show Search Area"=TRUE, "Show Search Lines"=TRUE, "Show Edges Found"=TRUE, "Show Result"=TRUE}, "ROI Descriptor"={"Global Rectangle"=[], "Contours"=[]}, "Process"=0}  # Analysis_Clamp_Parameter
        n17 = Variant To Data(type=w73, Variant=w74) -> (data=w70:T37)  [unwired: 1 in, 1 out]
        n18 = call "GetClampResultNames.vi"("ProjectName"=w72, "data"=w70, "ROI_Name"=w71) -> ("ResultNames"=w69:string[])  [unwired: 8 in]
      }
      frame 6 {
        w76 = T38 {"Overlay Settings"={"Show Search Area"=FALSE, "Show Curves"=FALSE, "Show Clamp Locations"=FALSE, "Show Result"=FALSE, "Search Area Color"=0, "Curves Color"=0, "Clamp Locations Color"=0, "Result Color"=0, "Overlay Group Name"=""}, "Curve Extraction Settings"={"Extraction Mode"=0, "Edge Threshold"=0, "Edge Filter Size"=0, "Min Length"=0, "Row Search Step Size"=0, "Col Search Step Size"=0, "Max Endpoint Gap"=0, "Closed"=FALSE, "Subpixel"=FALSE}, "Clamp Settings"={"Angle Range (+/-)"=0.0, "Edge Polarity"={"Start"=0, "End"=0}}, "ROI"={"Global Rectangle"=[], "Contours"=[]}}  # Analysis_Clamp MAX_Parameter
        n19 = Variant To Data(type=w76, Variant=w80) -> (data=w75:T38)  [unwired: 1 in, 1 out]
        n20 = call "GetClampMAXResultNames.vi"("ProjectName"=w79, "data"=w75, "ROI_Name"=w78) -> ("ResultNames"=w77:string[])  [unwired: 8 in]
      }
      frame 7 {
        w85 = T39 {"Selected Particle"=0, "Connectivity 4/8 (8)"=TRUE, "MaxParticle"=0}  # Analysis_Particle_Parameter
        n21 = Variant To Data(type="Selected Particle Report", Variant=w84) -> (data=w81:T1, error out=w82:errorcluster)  [unwired: 1 in]
        n22 = Variant To Data(type=w85, Variant=w90) -> (data=w86:T39)  [unwired: 1 in, 1 out]
        n23 = call <vilib>:"Clear Errors.vi"("error in (no error)"=w82) -> ()  [unwired: 5 in, 2 out]
        n24 = call "GetPirticleResultNames.vi"("ProjectName"=w89, "Selected Particle Report"=w81, "Analysis_Particle_Parameter"=w86, "ROI_Name"=w88) -> ("ResultNames"=w87:string[])  [unwired: 7 in]
      }
      frame 8 {
        w95 = T40 {"Interval Range"={"Minimum"=0.0, "Maximum"=0.0}, "ROI Out"={"Global Rectangle"=[], "Contours"=[]}, "Number of Classes"=256}  # Analysis_Histogram_Parameter
        n25 = Variant To Data(type=w95, Variant=w96) -> (data=w91:T40)  [unwired: 1 in, 1 out]
        n26 = call "GetHistoramResultNames.vi"("ProjectName"=w94, "Analysis_Histogram_Parameter"=w91, "ROI_Name"=w92) -> ("ResultNames"=w93:string[])  [unwired: 8 in]
      }
      frame 10 {
        n27 = Variant To Data(type=T10 {"ROI Descriptor"={"Global Rectangle"=[], "Contours"=[]}, "Options"={"Search  Direction"=0, "Edge Options"={"Edge Polarity"=0, "Kernel Size"=3, "Width"=3, "Minimum Edge Strength"=10.0, "Interpolation Type"=enum."Bilinear Fixed", "Data Processing Method"=enum."Average"}, "Show Search Area"=FALSE, "Show Search Lines"=FALSE, "Show Edges Found"=FALSE, "Show Result"=TRUE, "Search Area Color"=65280, "Search Lines Color"=255, "Edge Locations Color"=16776960, "Result Color"=16711680, "Overlay Group Name"=""}, "Circle Fit Options"={"Process"=enum."Get First Edge", "Step Size"=3.0, "Max Pixel Radius"=3}} ("Analysis_Circle_Parameter"), Variant=w102) -> (data=w98:T10)  [unwired: 1 in, 1 out]
        n28 = call "GetCircleResultNames.vi"("ProjectName"=w100, "Analysis_Circle_Parameter"=w98, "ROI_Name"=w99) -> ("ResultNames"=w97:string[])  [unwired: 8 in]
      }
      frame 9 {
        w103 = T41 {"ROI Descriptor"={"Global Rectangle"=[], "Contours"=[]}, "Number of Matches Requested"=1, "Edge Info Size"=0, "Options"={"Search Direction"=0, "Edge Options"={"Edge Polarity"=0, "Kernel Size"=4, "Width"=3, "Minimum Edge Strength"=1024.0, "Interpolation Type"=enum."Zero Order", "Data Processing Method"=enum."Median"}, "Show Search Area"=FALSE, "Show Search Lines"=FALSE, "Show Edges Found"=FALSE, "Show Result"=TRUE, "Search Area Color"=5, "Search Lines Color"=3, "Edge Locations Color"=50, "Result Color"=1, "Overlay Group Name"=""}, "Line Fit Options"={"Number of Lines"=0, "Type"=enum."Best Edge Rake", "Min. Score"=0.0, "Max. Score"=25.0, "Orientation"=5.0, "Angle Range"=45.0, "Angle Tolerance"=1.0, "Step Size"=7, "Min. SNR (db)"=0.0, "Min. Points (%)"=25.0, "Hough Iterations"=5}}  # Analysis_Find Straight Edge_Parameter
        n29 = Variant To Data(type=w103, Variant=w108) -> (data=w104:T41)  [unwired: 1 in, 1 out]
        n30 = call "GetStraight EdgeResultNames.vi"("ProjectName"=w105, "Analysis_Find Straight Edge_Parameter"=w104, "ROI_Name"=w107) -> ("ResultNames"=w106:string[])  [unwired: 8 in]
      }
      frame 11 {
        n31 = Variant To Data(type=T13 {"Enum_ShapeType"=enum."Circles", "MaxParticle"=1, "Descriptor"={"Set 1"=100.0, "Set 2"=10.0, "Set 3"=200.0, "Set 4"=10.0}, "Match Options"={"Rotation"=TRUE, "Scale"=FALSE, "Occlusion"=FALSE, "Range Settings"=[{"Match Constraints"=0, "Min"=0.0, "Max"=360.0}]}, "Curve Parameters"={"Extraction Mode"=0, "Edge Threshold"=75, "Edge Filter Size"=1, "Min Length"=25, "Row Search Step Size"=15, "Col Search Step Size"=15, "Max Endpoint Gap"=10, "Closed"=FALSE, "Subpixel"=FALSE}, " score"=500.0} ("SetParameter"), Variant=w114) -> (data=w110:T13)  [unwired: 1 in, 1 out]
        n32 = call "GetShapeResultNames.vi"("ProjectName"=w113, "SetParameter"=w110, "ROI_Name"=w112) -> ("ResultNames"=w109:string[])  [unwired: 8 in]
      }
      frame 12 {
        n33 = Variant To Data(type=T14 {"OCRSelectedLanaguage"=[]} ("OCR_Setting Parameter"), Variant=w118) -> (data=w116:T14)  [unwired: 1 in, 1 out]
        n34 = call "GetOCRResultName.vi"("ProjectName"=w120, "data"=w116, "ROI_Name"=w119) -> ("Array"=w115:string[])  [unwired: 7 in, 1 out]
      }
      frame 13 {
        n35 = call "GetContourResultName.vi"("ProjectName"=w122, "ROIName"=w123) -> ("ContourResultName"=w121:string[])  [unwired: 9 in]
      }
      frame 14 {
        n36 = Variant To Data(type=T15 {"Color Sensitivity"=0, "Learn Saturation Threshold"=80, "Minimum Match Score"=800.0, "Match Saturation Threshold"=80, "ROI Descriptor"={"Global Rectangle"=[], "Contours"=[]}, "TemplatePath"="", "ColorSpectrum"=[]} ("ColorMatchParameter"), Variant=w127) -> (data=w126:T15)  [unwired: 1 in, 1 out]
        n37 = Unbundle By Name(w126) -> ("ROI Descriptor.Contours"=w125:T44)
        n38 = Array Size(array=w125) -> (size(s)=w124:i32)
        n39 = for {
          N: w124 -> [_]
          tunnel: w131 -> [w135]
          tunnel: w130 -> [w134]
          tunnel: [w133] -> w129 mode=concatenating
          i -> [w132]
          n40 = call "GetColorMatchResultName.vi"("ProjectName"=w134, "Index"=w132, "ROIName"=w135) -> ("ContourResultName"=w133:string[])  [unwired: 8 in]
        }
      }
    }
    n41 = Build Array (concatenate)(w26, w24) -> (w25:string[])
  }
  n42 = call "UpdateCaliperToMainResultTable.vi"("Type"=enum16{"TagName", "Value"}."TagName", "ProjectName"="ProjectName") -> ("CaliperResultNames"=w4:string[])  [unwired: 9 in]
  n43 = property class="MCListbox (strict)"(reference="MCListbox Refnum") -> (reference out=w17:refnum<vi>, "ItemNames"=w15:string[][])  [unwired: 1 in, 1 out]
  n44 = Array Size(array=w15) -> (size(s)=w14:i32[])
  n45 = Index Array(array=w14) -> (element #1=w13:i32, element #2=w12:i32)  [unwired: 2 in]
  n46 = Equal To 0?(x=w13) -> (x = 0?=w11:bool)
  n47 = Equal To 0?(x=w12) -> (x = 0?=w10:bool)
  n48 = And(x=w11, y=w10) -> (x .and. y?=w9:bool)
  n49 = Build Array (concatenate)(w5, w4) -> (w3:string[])
  n50 = Array Size(array=w3) -> (size(s)=w8:i32)
  n51 = Equal To 0?(x=w8) -> (x = 0?=w7:bool)
  n52 = case shown="False" w9 {
    tunnel: w3 -> [w138 w148]
    tunnel: [w137 w147] -> w16
    tunnel: w15 -> [w136 _]
    tunnel: w7 -> [_ w146]
    frame False {
      n53 = disable-structure shown="Enabled" {
        disable-tunnel: w138 -> [w141 w145]
        disable-tunnel: [w140 w143] -> w137
        disable-tunnel: w136 -> [w139 _]
        frame Disabled {
          n54 = Replace Array Subset(array=w139, new element=w141, index (col)=0 ("disabled index (col)")) -> (w140:string[][])  [unwired: 1 in]
        }
        frame Enabled {
          n55 = Build Array(w145) -> (w144:string[][])
          n56 = Transpose 2D Array(2D array=w144) -> (transposed array=w143:string[][])
        }
      }
    }
    frame True {
      n57 = case shown="True" w146 {
        tunnel: w148 -> [w150 _]
        tunnel: [w149 string[][] []] -> w147
        frame False {
          n58 = Build Array(w150) -> (w151:string[][])
          n59 = Transpose 2D Array(2D array=w151) -> (transposed array=w149:string[][])
        }
        frame True {
        }
      }
    }
  }
  n60 = property class="MCListbox (strict)"(reference=w17, "ItemNames"=w16) -> ()  [unwired: 1 in, 2 out]
